vi "Mask Image ColorPlanes.vi"(0 "Rectangle":T2 {"Rotation" min=-90.0 max=90.0 step=1.0 format="%.2f"; "Left" scale=0.0..1024.0; "Right" scale=0.0..1024.0}, 1 "Image Model":T1, 5 "Image R/H":T1, 7 "Image G/S":T1, 9 "Image B/L":T1, 11 "error in (no error)":errorcluster, 12 "Filling Value (255)":i32=255, 14 "Background Value (0)":i32) -> (4 "R/HMasked_Image":T1, 6 "G/SMasked_Image":T1, 8 "B/LMasked_Image":T1, 15 "error out":errorcluster)   [LabVIEW 2017]
uses:
  <vilib>/vision/Image Controls.llb/IMAQ Image.ctl
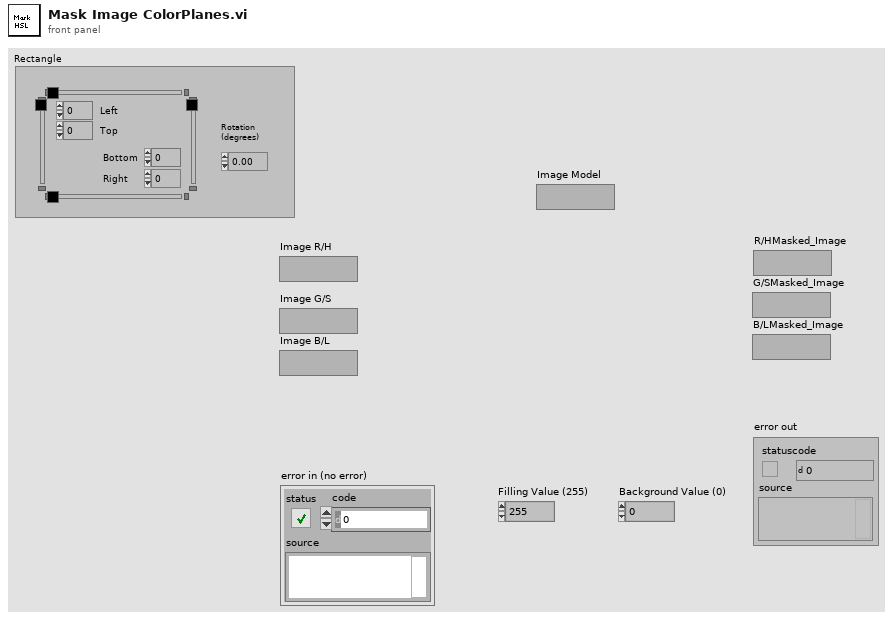
[diagram p1: front panel]
types:
  T1 = typedef "IMAQ Image.ctl" = refnum<image>
  T2 = typedef "IMAQ Rectangle" = cluster{"Left":i32, "Top":i32, "Right":i32, "Bottom":i32, "Rotation":dbl}
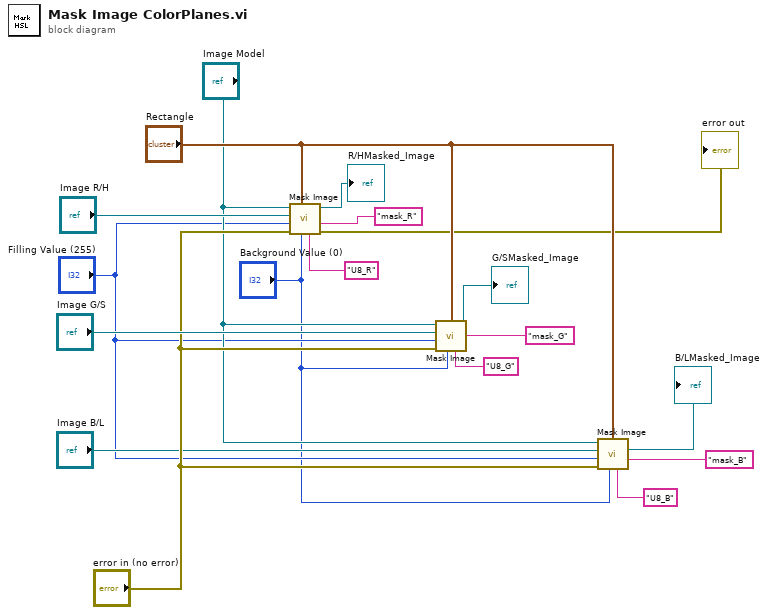
[diagram p0: block diagram]
diagram:
  n1 = call "Mask Image.vi"("Image Name Out"="mask_R", "Image Name"="U8_R", "Background Value (0)"="Background Value (0)", "Rectangle"="Rectangle", "error in (no error)"="error in (no error)", "Filling Value (255)"="Filling Value (255)", "Image Src"="Image R/H", "Image Model"="Image Model") -> ("error out"=→"error out":errorcluster, "Masked_Image"=→"R/HMasked_Image":T1)  [unwired: 1 in, 1 out]
  n2 = call "Mask Image.vi"("Image Name Out"="mask_G", "Image Name"="U8_G", "Background Value (0)"="Background Value (0)", "Rectangle"="Rectangle", "error in (no error)"="error in (no error)", "Filling Value (255)"="Filling Value (255)", "Image Src"="Image G/S", "Image Model"="Image Model") -> ("Masked_Image"=→"G/SMasked_Image":T1)  [unwired: 1 in, 2 out]
  n3 = call "Mask Image.vi"("Image Name Out"="mask_B", "Image Name"="U8_B", "Background Value (0)"="Background Value (0)", "Rectangle"="Rectangle", "error in (no error)"="error in (no error)", "Filling Value (255)"="Filling Value (255)", "Image Src"="Image B/L", "Image Model"="Image Model") -> ("Masked_Image"=→"B/LMasked_Image":T1)  [unwired: 1 in, 2 out]
